vi "Stop.vi"(8 "error in (no error)":errorcluster, 11 "reference in":refnum<class "mmWave instrument.lvclass">) -> (0 "error out":errorcluster, 3 "reference out":refnum<class "mmWave instrument.lvclass">)   [LabVIEW 2019, in "mmWave instrument.lvclass"]
doc: "Stop operation"
uses:
  mmWave instrument.lvclass
  Instrument state.ctl
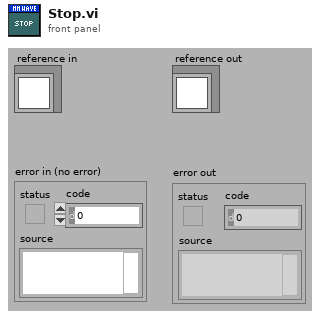
[diagram p1: front panel]
types:
  T1 = typedef "mmWave instrument.lvclass/Instrument state.ctl" = enum16{"Off", "Initialization", "Configuration", "Running", "Calibration"}
  T2 = typedef "mmWave instrument.lvclass/ObjectAttributes.ctl" = cluster{"mode":T3, "instr state":T1, "Max Fs":dbl, "Equalization coeff":cdb[], "LO sync en":bool, "Trig sync en":bool, "LO sources":T4, "LO Export":T5, "Fc.range":cluster{"min":dbl, "max":dbl}, "Sync mode":T6, "equalization en":bool, "sequence":string[]}
  T3 = typedef "mmWave instrument.lvclass/Instrument mode.ctl" = enum16{"RF", "IF", "BB"}
  T4 = typedef "mmWave HW Control.lvlib/LO sources.ctl" = cluster{"RX/LO1 src":string, "TX/LO1 src":string, "LO2 src":string}
  T5 = typedef "mmWave HW Control.lvlib/LO export.ctl" = cluster{"TX LO1 export":bool, "TX LO1 export level":dbl, "RX LO1 export":bool, "RX LO1 export level":dbl, "LO2 export":bool, "LO2 export level":dbl}
  T6 = typedef "mmWave instrument.lvclass/Sync mode.ctl" = enum16{"Slave", "Master"}
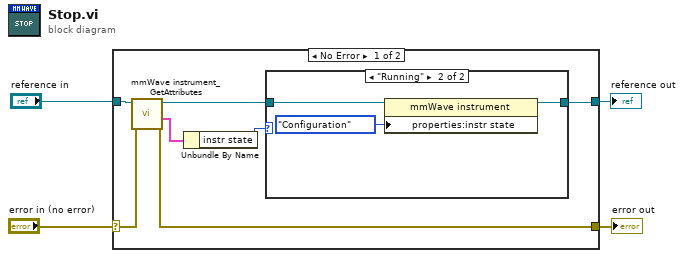
[diagram p0: block diagram]
diagram:
  n1 = case shown="No Error" "error in (no error)" {
    selector: "error in (no error)" -> [w11 w17]
    tunnel: [w10 w17] -> w3
    tunnel: [w5 w16] -> w1
    tunnel: "reference in" -> [w8 w16]
    frame No Error {
      n2 = call "mmWave instrument_GetAttributes.vi"("error in (no error)"=w11, "reference in"=w8) -> ("error out"=w10:errorcluster, "attributes"=w9:T2, "reference out"=w7:refnum<class "mmWave instrument.lvclass">)  [unwired: 6 in, 1 out]
      n3 = Unbundle By Name(w9) -> ("instr state"=w6:T1)
      n4 = case shown="\"Running\"" w6 {
        tunnel: w7 -> [w12 w15]
        tunnel: [w12 w14] -> w5
        frame "Off", Default {
        }
        frame "Running" {
          n5 = property class="mmWave instrument"(reference=w15, "properties:instr state"=Instrument_state."Configuration" ("instr state")) -> (reference out=w14:refnum<class "mmWave instrument.lvclass">)  [unwired: 1 in, 1 out]
        }
      }
    }
    frame Error {
    }
  }
  "error out" <- w3
  "reference out" <- w1
